vi "Applied Send Command.vi"(6 "error in (no error)":errorcluster, 7 "Extra":string, 8 "Command":T1(ring), 9 "VISA resource name":refnum<visa-resource-name>="COM1") -> (0 "error out":errorcluster, 2 "read buffer":string, 3 "VISA resource name out":refnum<visa-resource-name>)   [LabVIEW 2015]
uses:
  Instance           1 28Saved   Applied Send Command .vi
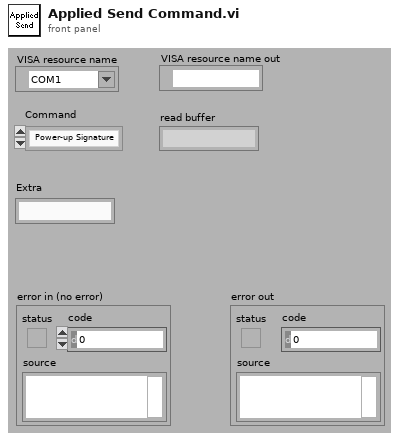
[diagram p1: front panel]
types:
  T1 = enum16{"Power-up Signature", "Accel Rate", "Accel Max", "Bit Rate", "Buffer Status", "Change Current", "Commence Jogging", "Change Jog Speed", "Continue", "Define Address", "Distance for FC,FM,FO,FY", "Decel Rate", "Distance or Position", "Define Limits", "Encoder Deadband", "Encoder Function", "Encoder Position", "Encoder Ratio", "Feed to Length with Speed Change", "Feed to Length", "Feed to Sensor with Mask Dist", "Feed to Length & Set Output", "Feed to Position", "Feed to Sensor", "Feed to Sensor w/safety", "Follow Handwheel", "Immediate Distance?", "Immediate Encoder?", "Immediate Low Output", "Immediate High Output", "Immediate Position?", "Input Status?", "Jog Accel/Decel", "Jog Disable", "Jog Enable", "Jog Speed", "Motor Disable", "Motor Enable", "Microstep Resolution", "Power up Current", "Power up Mode", "Pause", "Request Status", "Revision Level?", "Seek Home", "Stop Jogging", "Stop & Kill Buffer", "Set Output", "Set ABS Position", "Send String", "Stop", "Velocity for Speed Change", "Velocity Setting", "Wait for Input", "Wait Time"}
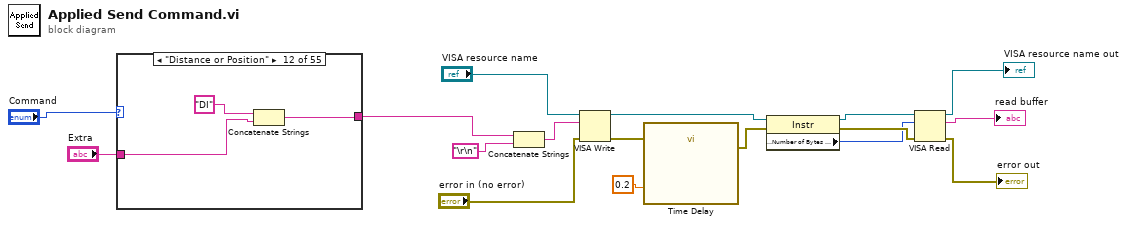
[diagram p0: block diagram]
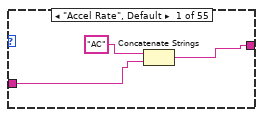
[diagram p2: hidden frame]
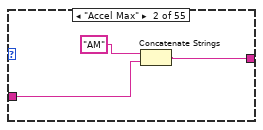
[diagram p3: hidden frame]
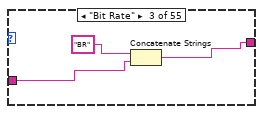
[diagram p4: hidden frame]
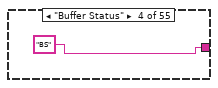
[diagram p5: hidden frame]
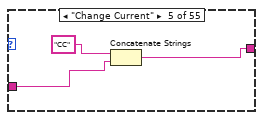
[diagram p6: hidden frame]
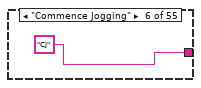
[diagram p7: hidden frame]
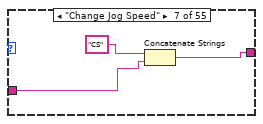
[diagram p8: hidden frame]
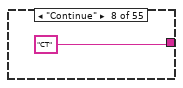
[diagram p9: hidden frame]
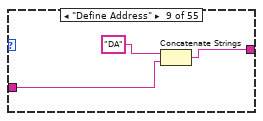
[diagram p10: hidden frame]
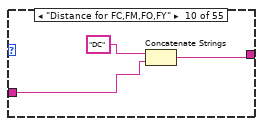
[diagram p11: hidden frame]
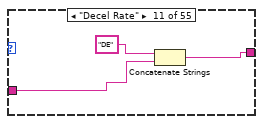
[diagram p12: hidden frame]
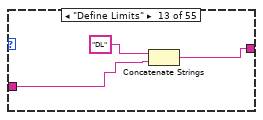
[diagram p13: hidden frame]
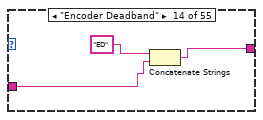
[diagram p14: hidden frame]
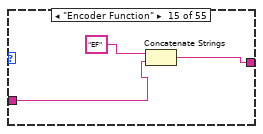
[diagram p15: hidden frame]
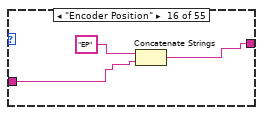
[diagram p16: hidden frame]
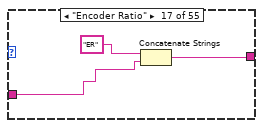
[diagram p17: hidden frame]
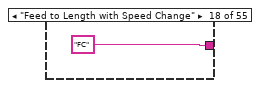
[diagram p18: hidden frame]
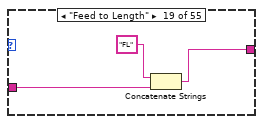
[diagram p19: hidden frame]
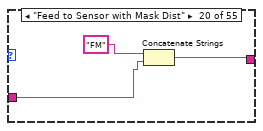
[diagram p20: hidden frame]
diagram:
  n1 = case shown="\"Distance or Position\"" "Command" {
    tunnel: "Extra" -> [w18 w22 w24 _ w28 _ w32 _ w36 w39 w42 w45 w49 w51 w54 w57 w60 _ w64 w67 w70 w73 w76 w79 w82 _ _ w87 w90 _ _ w95 _ _ w100 _ _ w105 w108 w111 _ _ _ w117 _ _ w122 w125 w128 _ w132 w136 w138 w141 _]
    tunnel: [w19 w21 w25 "BS" w29 "CJ" w33 "CT" w37 w40 w43 w46 w48 w52 w55 w58 w61 "FC" w65 w68 w71 w74 w77 w80 w83 "ID" "IE" w88 w91 "IP" "IS" w96 "JD" "JE" w101 "CT" "ME" w106 w109 w112 "PS" "RS" "RV" w118 "SJ" "SK" w123 w126 w129 "ST" w133 w135 w139 w142 "00"] -> w2
    frame "Accel Rate", Default {
      n2 = Concatenate Strings("AC", w18) -> (w19:string)
    }
    frame "Accel Max" {
      n3 = Concatenate Strings("AM", w22) -> (w21:string)
    }
    frame "Bit Rate" {
      n4 = Concatenate Strings("BR", w24) -> (w25:string)
    }
    frame "Buffer Status" {
    }
    frame "Change Current" {
      n5 = Concatenate Strings("CC", w28) -> (w29:string)
    }
    frame "Commence Jogging" {
    }
    frame "Change Jog Speed" {
      n6 = Concatenate Strings("CS", w32) -> (w33:string)
    }
    frame "Continue" {
    }
    frame "Define Address" {
      n7 = Concatenate Strings("DA", w36) -> (w37:string)
    }
    frame "Distance for FC,FM,FO,FY" {
      n8 = Concatenate Strings("DC", w39) -> (w40:string)
    }
    frame "Decel Rate" {
      n9 = Concatenate Strings("DE", w42) -> (w43:string)
    }
    frame "Distance or Position" {
      n10 = Concatenate Strings("DI", w45) -> (w46:string)
    }
    frame "Define Limits" {
      n11 = Concatenate Strings("DL", w49) -> (w48:string)
    }
    frame "Encoder Deadband" {
      n12 = Concatenate Strings("ED", w51) -> (w52:string)
    }
    frame "Encoder Function" {
      n13 = Concatenate Strings("EF", w54) -> (w55:string)
    }
    frame "Encoder Position" {
      n14 = Concatenate Strings("EP", w57) -> (w58:string)
    }
    frame "Encoder Ratio" {
      n15 = Concatenate Strings("ER", w60) -> (w61:string)
    }
    frame "Feed to Length with Speed Change" {
    }
    frame "Feed to Length" {
      n16 = Concatenate Strings("FL", w64) -> (w65:string)
    }
    frame "Feed to Sensor with Mask Dist" {
      n17 = Concatenate Strings("FM", w67) -> (w68:string)
    }
    frame "Feed to Length & Set Output" {
      n18 = Concatenate Strings("FO", w70) -> (w71:string)
    }
    frame "Feed to Position" {
      n19 = Concatenate Strings("FP", w73) -> (w74:string)
    }
    frame "Feed to Sensor" {
      n20 = Concatenate Strings("FS", w76) -> (w77:string)
    }
    frame "Feed to Sensor w/safety" {
      n21 = Concatenate Strings("FY", w79) -> (w80:string)
    }
    frame "Follow Handwheel" {
      n22 = Concatenate Strings("HW", w82) -> (w83:string)
    }
    frame "Immediate Distance?" {
    }
    frame "Immediate Encoder?" {
    }
    frame "Immediate Low Output" {
      n23 = Concatenate Strings("IL", w87) -> (w88:string)
    }
    frame "Immediate High Output" {
      n24 = Concatenate Strings("IH", w90) -> (w91:string)
    }
    frame "Immediate Position?" {
    }
    frame "Input Status?" {
    }
    frame "Jog Accel/Decel" {
      n25 = Concatenate Strings("JA", w95) -> (w96:string)
    }
    frame "Jog Disable" {
    }
    frame "Jog Enable" {
    }
    frame "Jog Speed" {
      n26 = Concatenate Strings("JS", w100) -> (w101:string)
    }
    frame "Motor Disable" {
    }
    frame "Motor Enable" {
    }
    frame "Microstep Resolution" {
      n27 = Concatenate Strings("MR", w105) -> (w106:string)
    }
    frame "Power up Current" {
      n28 = Concatenate Strings("PC", w108) -> (w109:string)
    }
    frame "Power up Mode" {
      n29 = Concatenate Strings("PM", w111) -> (w112:string)
    }
    frame "Pause" {
    }
    frame "Request Status" {
    }
    frame "Revision Level?" {
    }
    frame "Seek Home" {
      n30 = Concatenate Strings("SH", w117) -> (w118:string)
    }
    frame "Stop Jogging" {
    }
    frame "Stop & Kill Buffer" {
    }
    frame "Set Output" {
      n31 = Concatenate Strings("SO", w122) -> (w123:string)
    }
    frame "Set ABS Position" {
      n32 = Concatenate Strings("SP", w125) -> (w126:string)
    }
    frame "Send String" {
      n33 = Concatenate Strings("SS", w128) -> (w129:string)
    }
    frame "Stop" {
    }
    frame "Velocity for Speed Change" {
      n34 = Concatenate Strings("VC", w132) -> (w133:string)
    }
    frame "Velocity Setting" {
      n35 = Concatenate Strings("VE", w136) -> (w135:string)
    }
    frame "Wait for Input" {
      n36 = Concatenate Strings("WI", w138) -> (w139:string)
    }
    frame "Wait Time" {
      n37 = Concatenate Strings("WT", w141) -> (w142:string)
    }
    frame "Power-up Signature" {
    }
  }
  n38 = Concatenate Strings(w2, "\r\n") -> (w10:string)
  n39 = VISA Write(VISA resource name="VISA resource name", write buffer=w10, error in (no error)="error in (no error)") -> (VISA resource name out=w17:refnum<visa-resource-name>, error out=w8:errorcluster)  [unwired: 1 out]
  n40 = call "Time Delay"("error in (no error)"=w8, "Delay Time (s)"=0.2) -> ("error out"=w7:errorcluster)  [unwired: 9 in]
  n41 = property class="Instr"(reference=w17, error in=w7) -> (reference out=w15:refnum<visa-resource-name>, error out=w16:errorcluster, "Serial Settings:Number of Bytes at Serial Port"=w14:u32)
  n42 = VISA Read(VISA resource name=w15, byte count=w14, error in (no error)=w16) -> (VISA resource name out=→"VISA resource name out":refnum<visa-resource-name>, read buffer=→"read buffer":string, error out=→"error out":errorcluster)  [unwired: 1 out]
